vi "Scan all possible zip extention case combos.vi"(11 "Path containing Zipped files":path) -> (0 "error out":errorcluster, 3 "Zipped Files List":string[](array[string]))   [LabVIEW 2012]
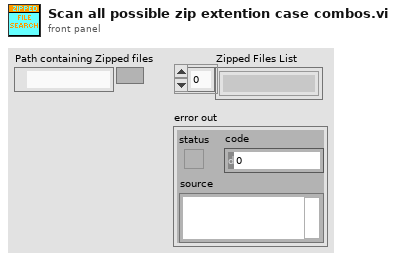
[diagram p1: front panel]
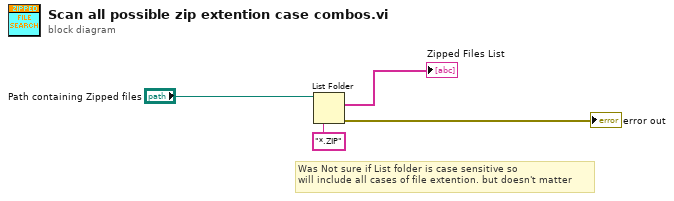
[diagram p0: block diagram]
diagram:
  # "Was Not sure if List folder is case sensitive so\nwill include all cases of file extention. but doesn't matter"
  n1 = List Folder(path="Path containing Zipped files", pattern="*.ZIP") -> (filenames=→"Zipped Files List":string[], error out=→"error out":errorcluster)  [unwired: 2 in, 2 out]
